vi "test Read XY from Tag To ClusterArray.vi"(8 "error in (no error)":errorcluster, 11 "TestCase in":refnum<class "Utility VIs tests.lvclass">) -> (0 "error out":errorcluster, 3 "TestCase out":refnum<class "Utility VIs tests.lvclass">)   [LabVIEW 2014, in "Utility VIs tests.lvclass"]
uses:
  Utility VIs tests.lvclass
  <vilib>/addons/_JKI Toolkits/VI Tester/TestCase.llb/TestCase.lvclass
  SPLAT/Tag.lvclass
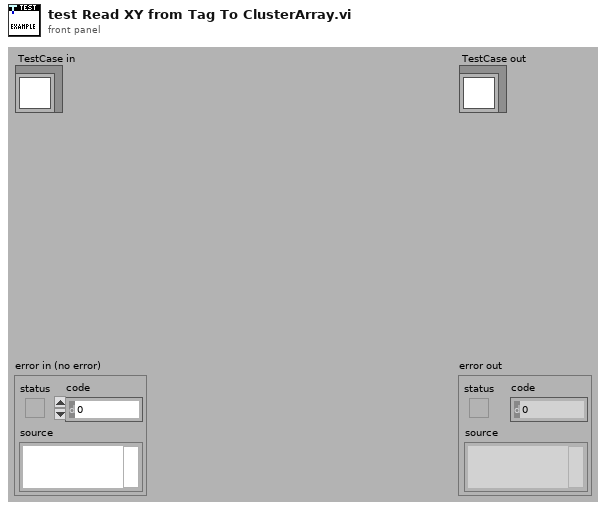
[diagram p1: front panel]
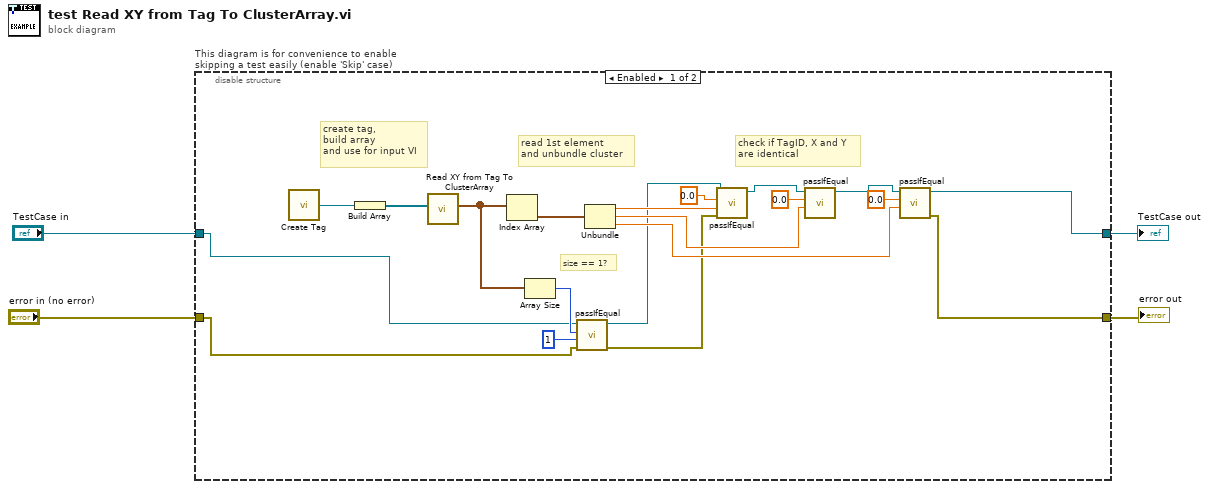
[diagram p0: block diagram]
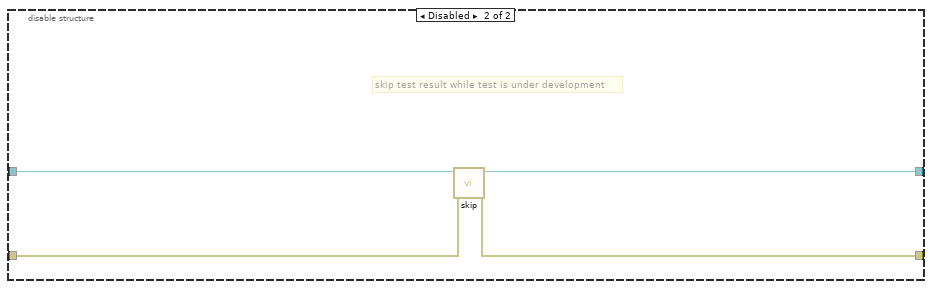
[diagram p2: hidden frame]
diagram:
  n1 = disable-structure "This diagram is for convenience to enable skipping a test easily (enable 'Skip' case)" shown="Enabled" {
    disable-tunnel: "TestCase in" -> [w18 w28]
    disable-tunnel: [w6 w26] -> w1
    disable-tunnel: [w5 w27] -> w3
    disable-tunnel: "error in (no error)" -> [w17 w25]
    frame Enabled {
      # "size == 1?"
      # "check if TagID, X and Y\nare identical"
      # "read 1st element\nand unbundle cluster"
      # "create tag,\nbuild array\nand use for input VI"
      n2 = call "Create Tag.vi"() -> ("Tag Out"=w24:refnum<class "Tag.lvclass">)  [unwired: 3 in]
      n3 = Build Array(w24) -> (w23:refnum<class "Tag.lvclass">[])
      n4 = call "Read XY from Tag To ClusterArray.vi"("Input TagArray"=w23) -> ("Tag ClusterArray Out"=w21:cluster{"TagID":dbl, "TagX":dbl, "TagY":dbl}[])  [unwired: 10 in]
      n5 = Index Array(array=w21) -> (element=w22:cluster{"TagID":dbl, "TagX":dbl, "TagY":dbl})  [unwired: 1 in]
      n6 = Array Size(array=w21) -> (size(s)=w20:i32)
      n7 = call-dynamic "passIfEqual.vi"("error in (no error)"=w17, "y"=1, "x"=w20, "TestCase in"=w18) -> ("error out"=w8:errorcluster, "TestCase out"=w11:refnum<class "Utility VIs tests.lvclass">)  [unwired: 6 in]
      n8 = Unbundle(w22) -> ("TagID"=w16:dbl, "TagX"=w15:dbl, "TagY"=w14:dbl)
      n9 = call-dynamic "passIfEqual.vi"("error in (no error)"=w8, "y"=w16, "x"=0.0, "TestCase in"=w11) -> ("TestCase out"=w10:refnum<class "Utility VIs tests.lvclass">)  [unwired: 6 in, 1 out]
      n10 = call-dynamic "passIfEqual.vi"("y"=w15, "x"=0.0, "TestCase in"=w10) -> ("TestCase out"=w9:refnum<class "Utility VIs tests.lvclass">)  [unwired: 7 in, 1 out]
      n11 = call-dynamic "passIfEqual.vi"("y"=w14, "x"=0.0, "TestCase in"=w9) -> ("error out"=w5:errorcluster, "TestCase out"=w6:refnum<class "Utility VIs tests.lvclass">)  [unwired: 7 in]
    }
    frame Disabled {
      # "skip test result while test is under development"
      n12 = call <vilib>:"skip.vi"("error in (no error)"=w25, "TestCase in"=w28) -> ("error out"=w27:errorcluster, "TestCase out"=w26:refnum<class "Utility VIs tests.lvclass">)  [unwired: 8 in]
    }
  }
  "error out" <- w3
  "TestCase out" <- w1
